vi "GLVT-Main.vi"() -> ()   [LabVIEW 2020]
uses:
  Controls/GLVT-States.ctl
  Controls/GLVT-Stepper-EnableState.ctl
  Controls/GLVT-Stepper-RotateDirection.ctl
  <vilib>/numeric/Random Number (Range) DBL.vi
  Controls/GLVT-FGV-States.ctl
panel:
  out "Filename DTS":string
  out "Save Data Location":path
  in  "Filename Descriptor":string
  out "End Data Collection":bool
  out "Current Angle Array Location":i32
  out "Working":bool
  in  "Measure Valve Button":bool
  out "Collected Data":cluster{dbl[], dbl[]}(graph)
  out "Angles for Data Collection (deg abs)":dbl[](array[numeric])
  in  "Angle per Step":dbl=1.0 min=1.0 step=0.1
  in  "Max Angle to Rotate (deg abs)":dbl
  in  "Pulse Rate (pps)":i32=600
  in  "Steps per Rev":i32=1600
  in  "Move Stepper Button":bool
  in  "Angle to Rotate  (deg abs)":dbl step=0.1
  out "Motor Position Actual":dbl format="%#.2f"
  in  "Release Motor Button":bool
  in  "Motor State":T1
  # "Configuration Only\nDo Not Change"
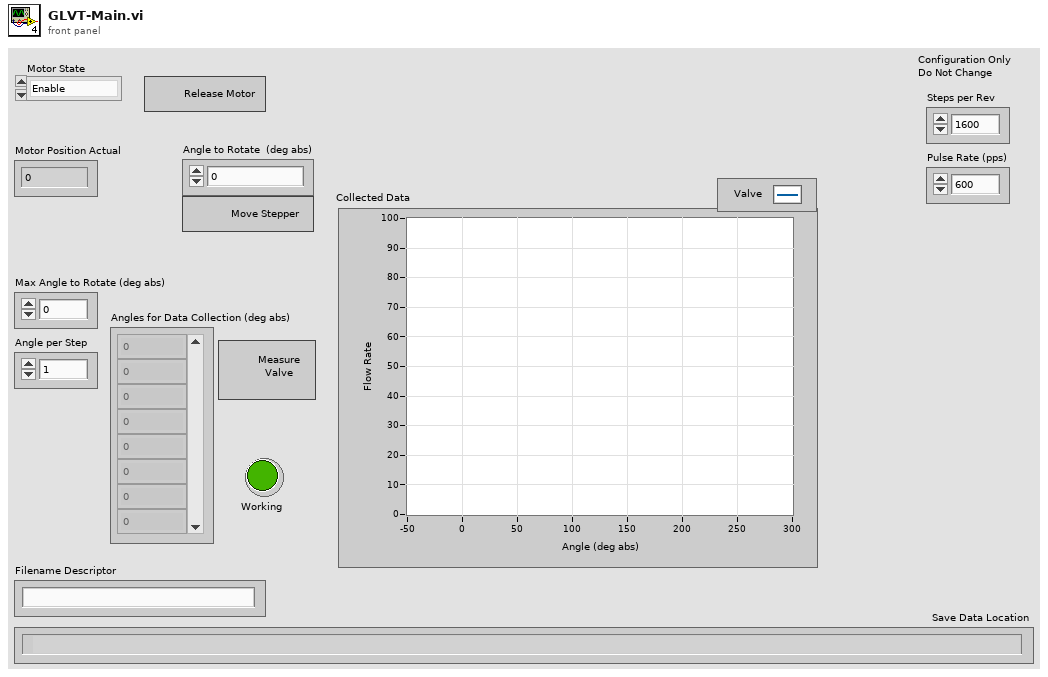
[diagram p1: front panel]
types:
  T1 = typedef "GLVT-Stepper-EnableState.ctl" = enum16{"Enable", "Disable"}
  T2 = typedef "GLVT-States.ctl" = enum16{"Idle", "Initialize", "Read Data", "Next Valve Pos", "Rotate Valve", "Save Data", "Exit"}
  T3 = typedef "GLVT-Stepper-RotateDirection.ctl" = enum16{"CCW", "CW"}
  T4 = typedef "GLVT-FGV-States.ctl" = enum16{"Get", "Set"}
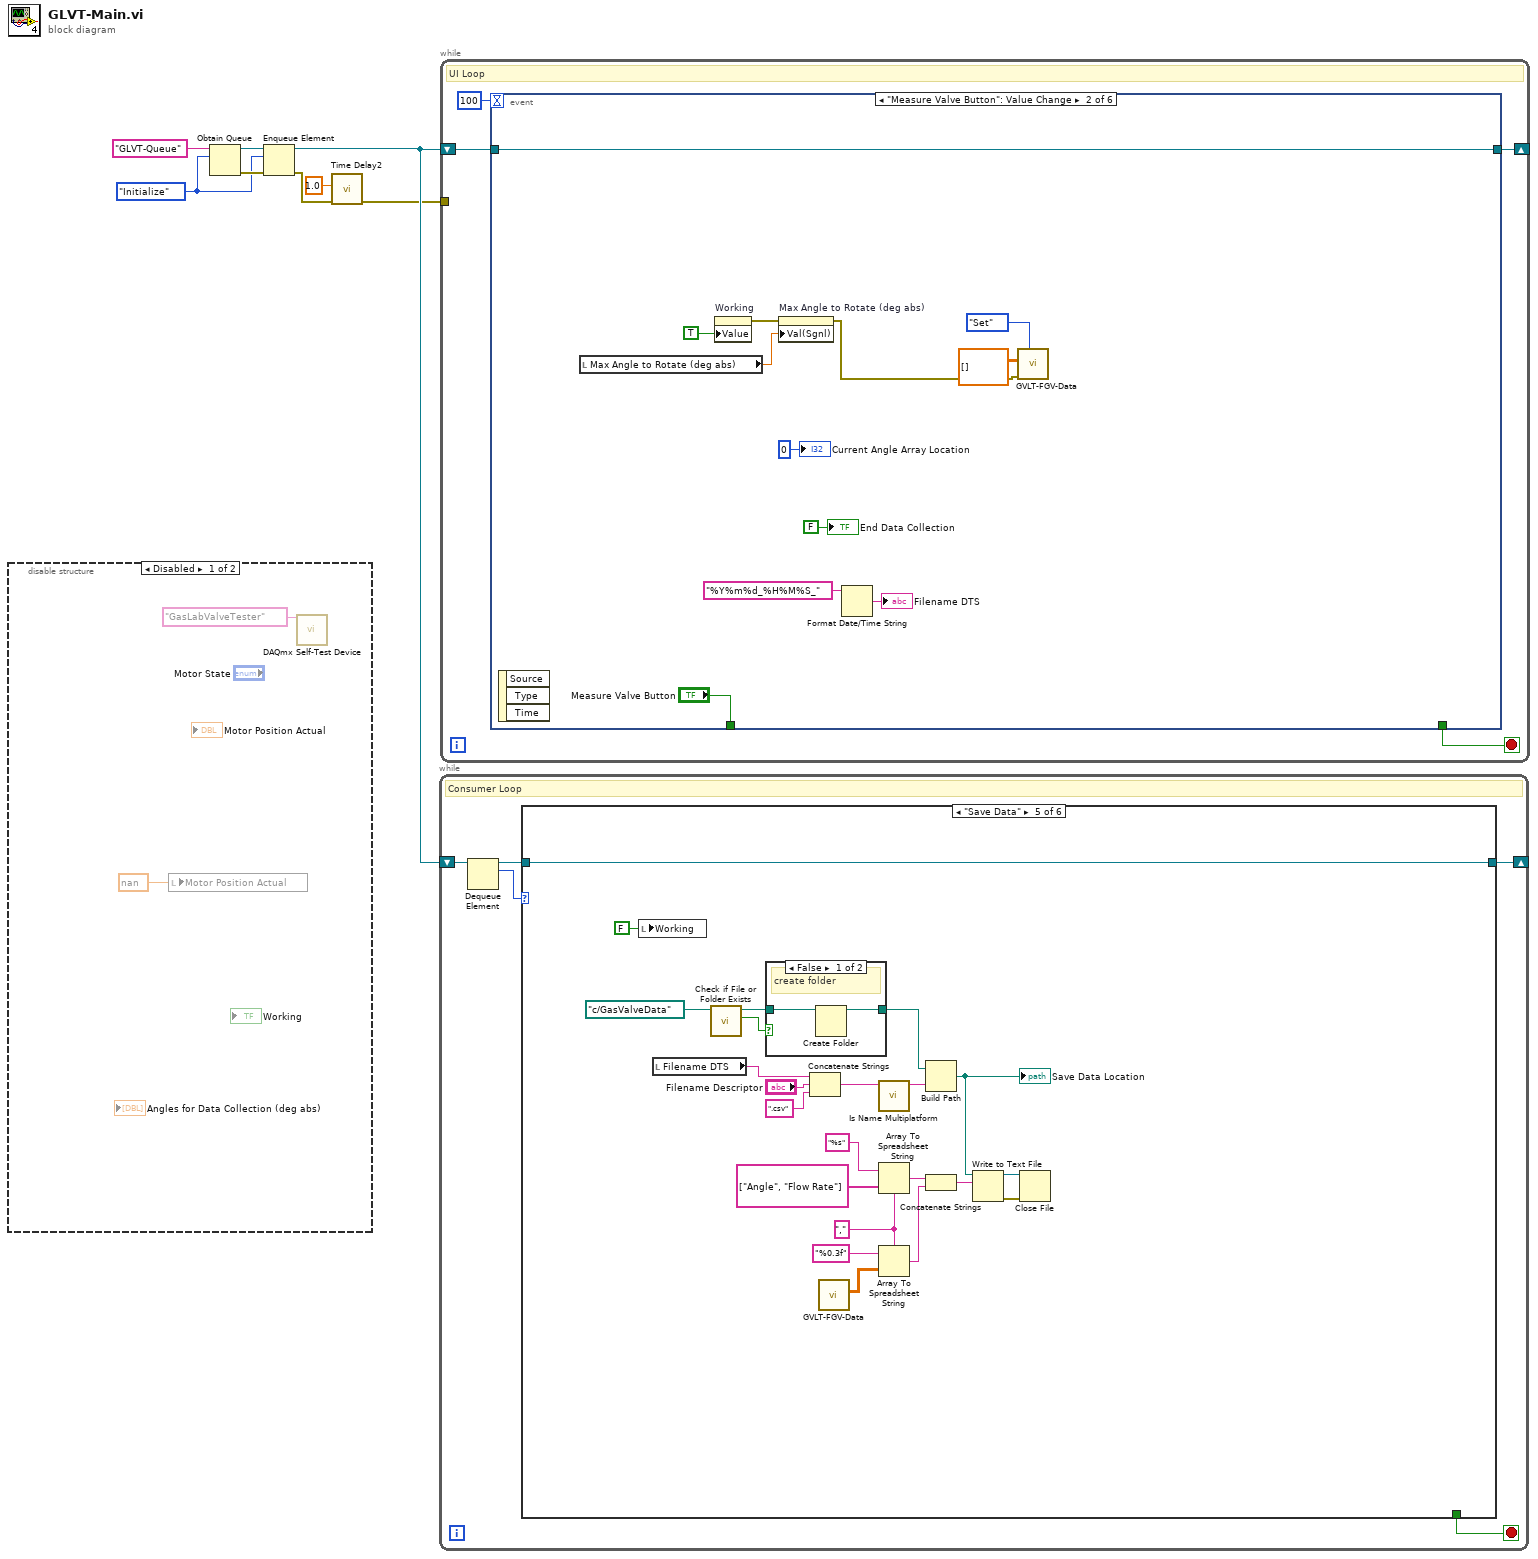
[diagram p0: block diagram]
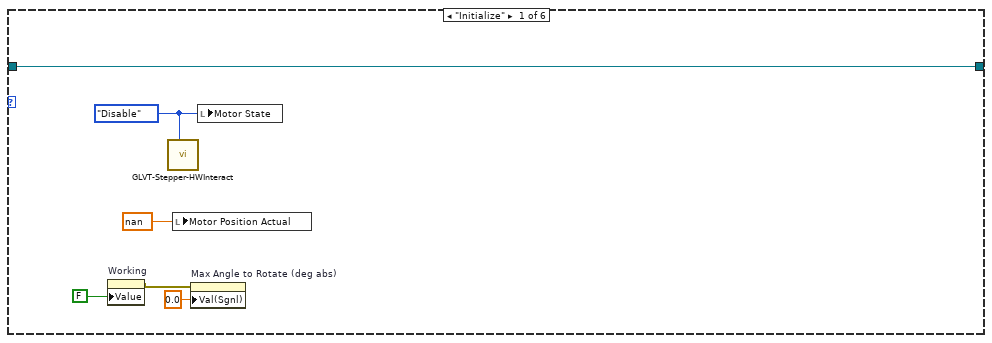
[diagram p3: hidden frame]
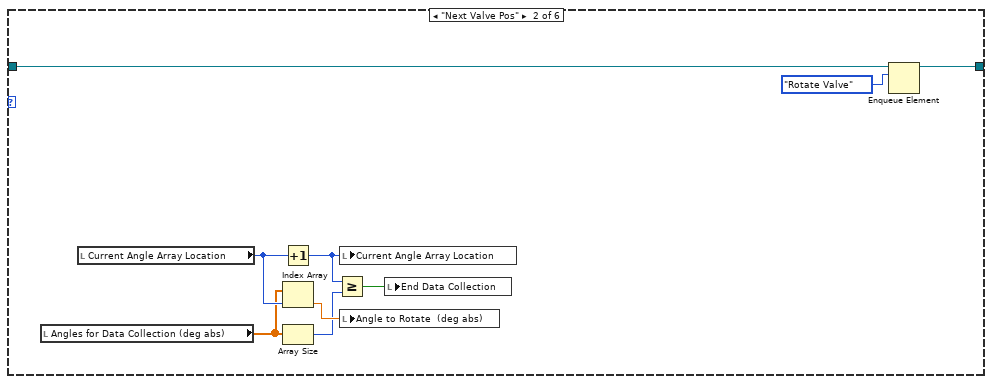
[diagram p4: hidden frame]
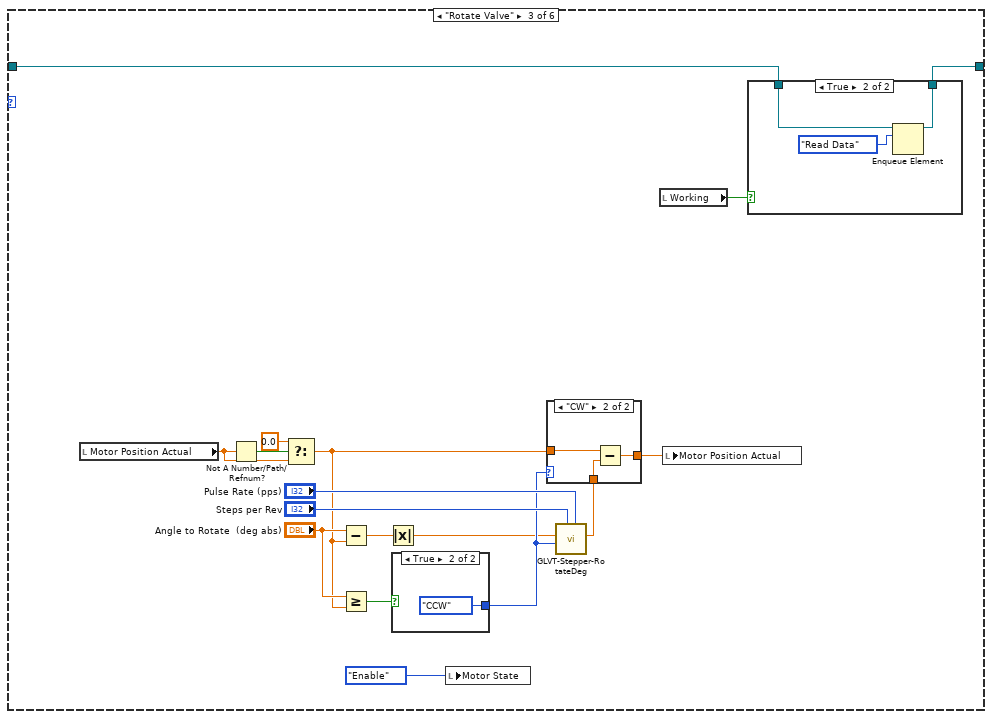
[diagram p5: hidden frame]
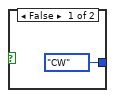
[diagram p7: hidden frame]
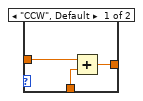
[diagram p8: hidden frame]
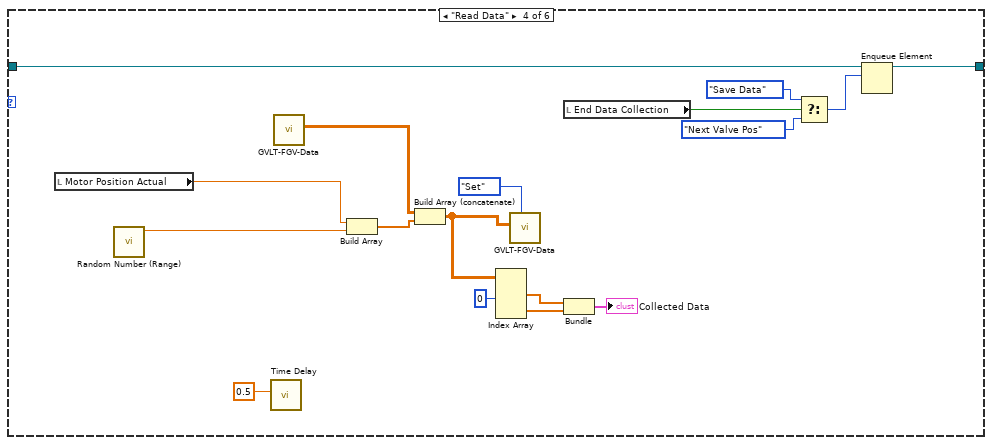
[diagram p9: hidden frame]
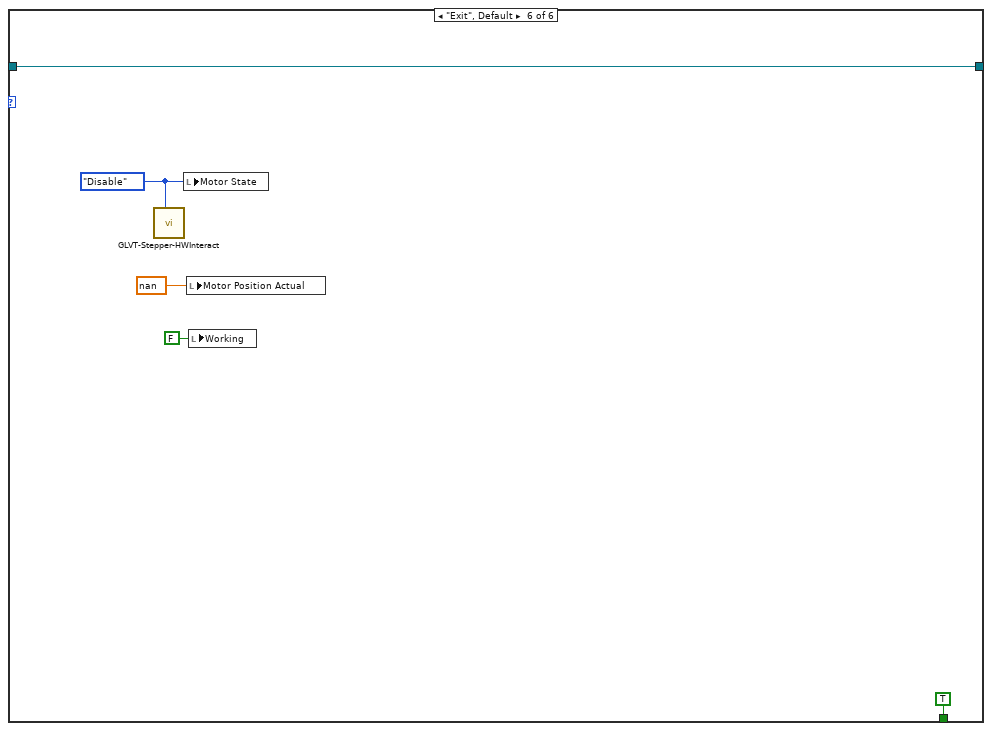
[diagram p11: hidden frame]
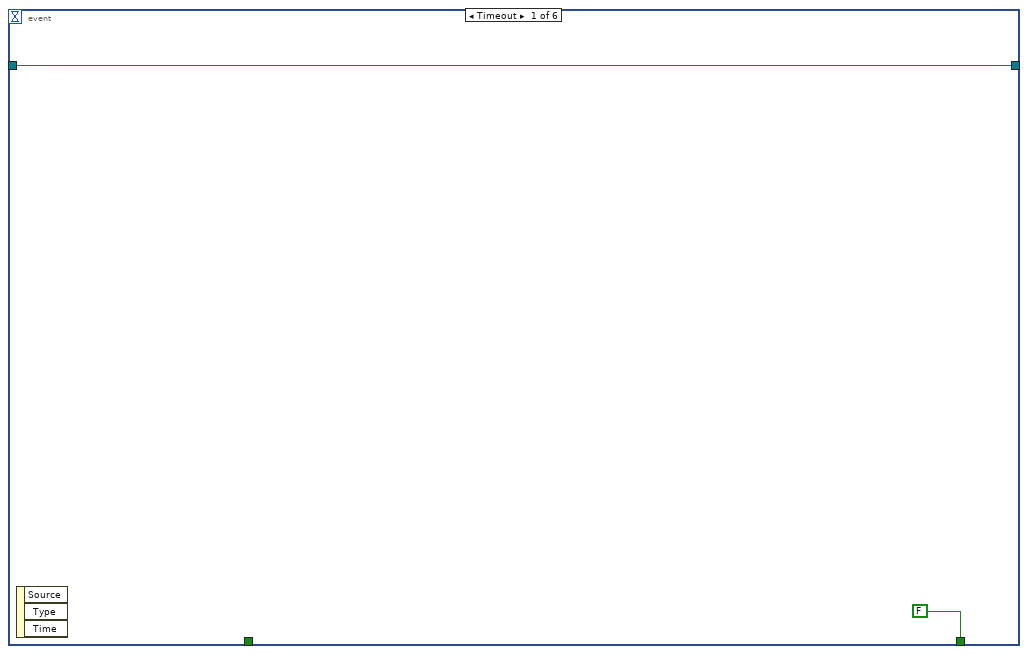
[diagram p12: hidden frame]
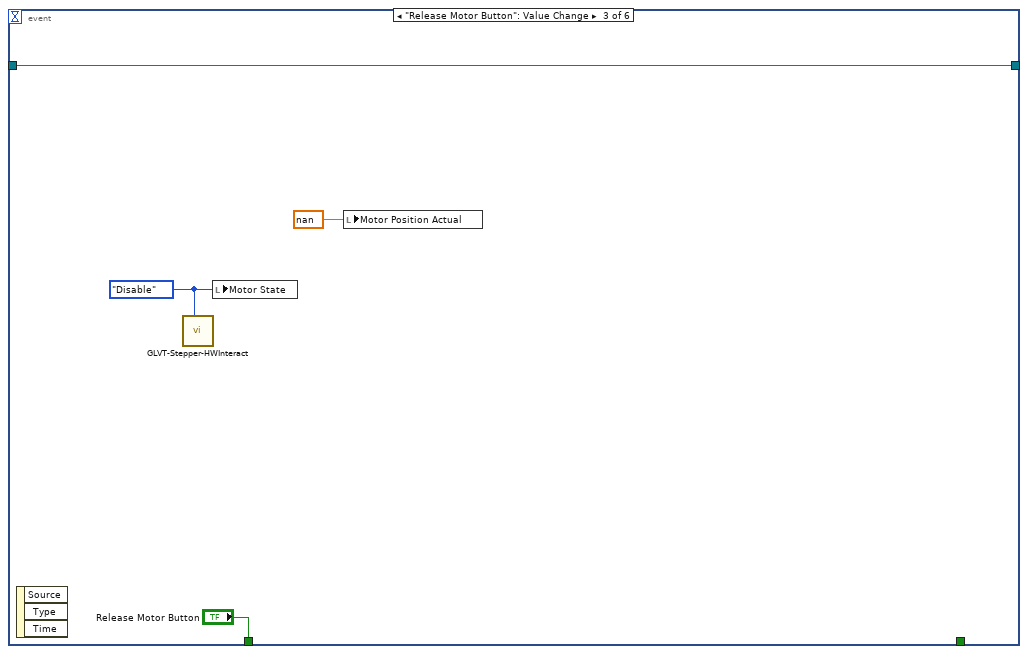
[diagram p13: hidden frame]
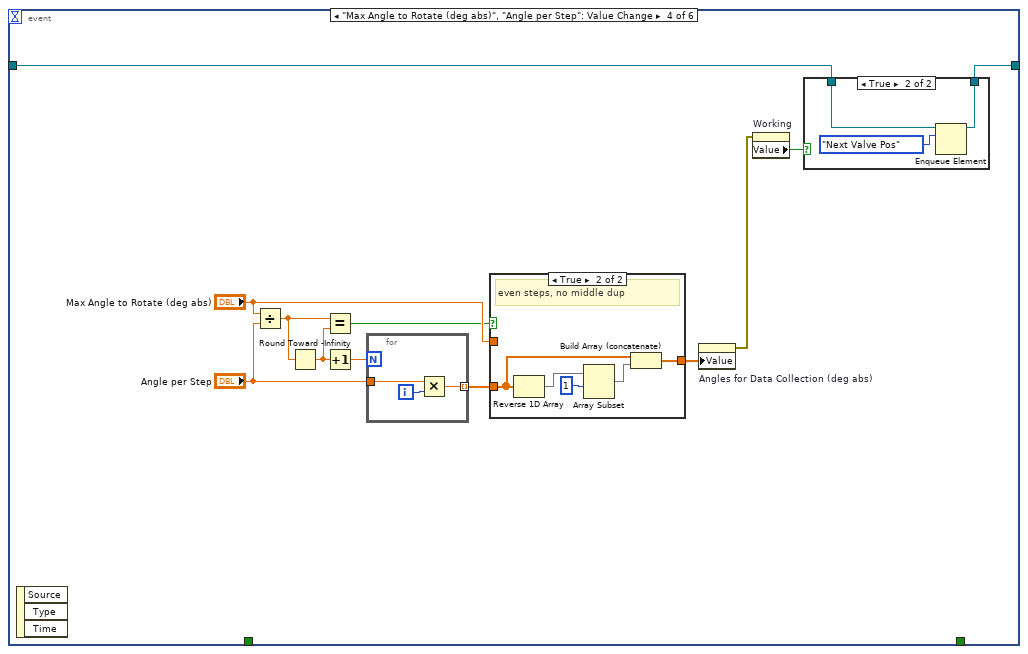
[diagram p14: hidden frame]
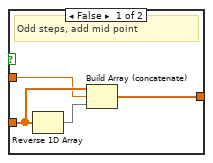
[diagram p16: hidden frame]
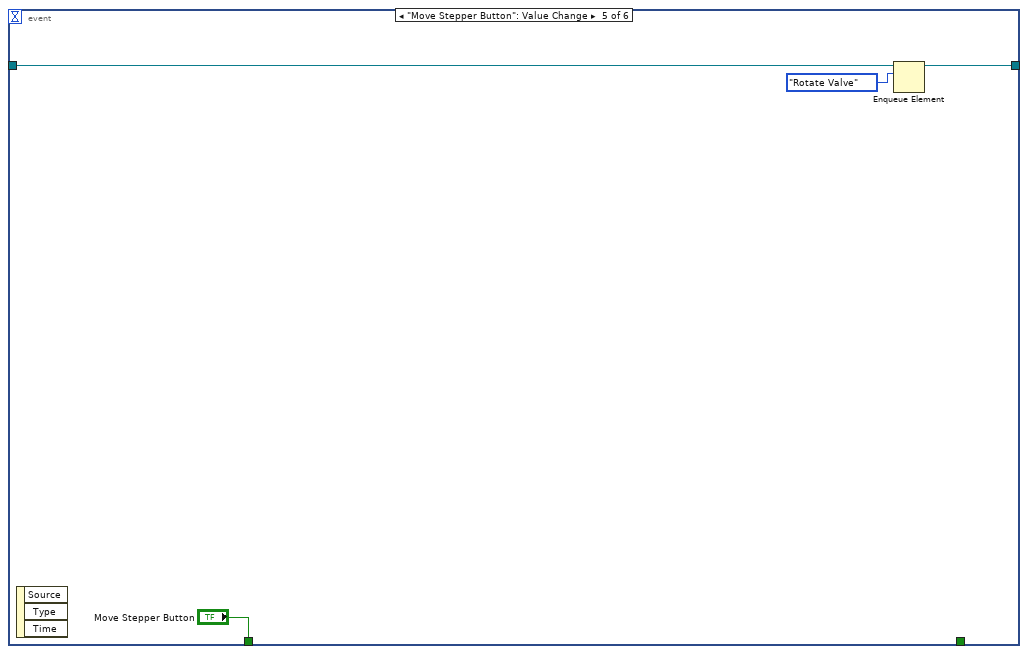
[diagram p17: hidden frame]
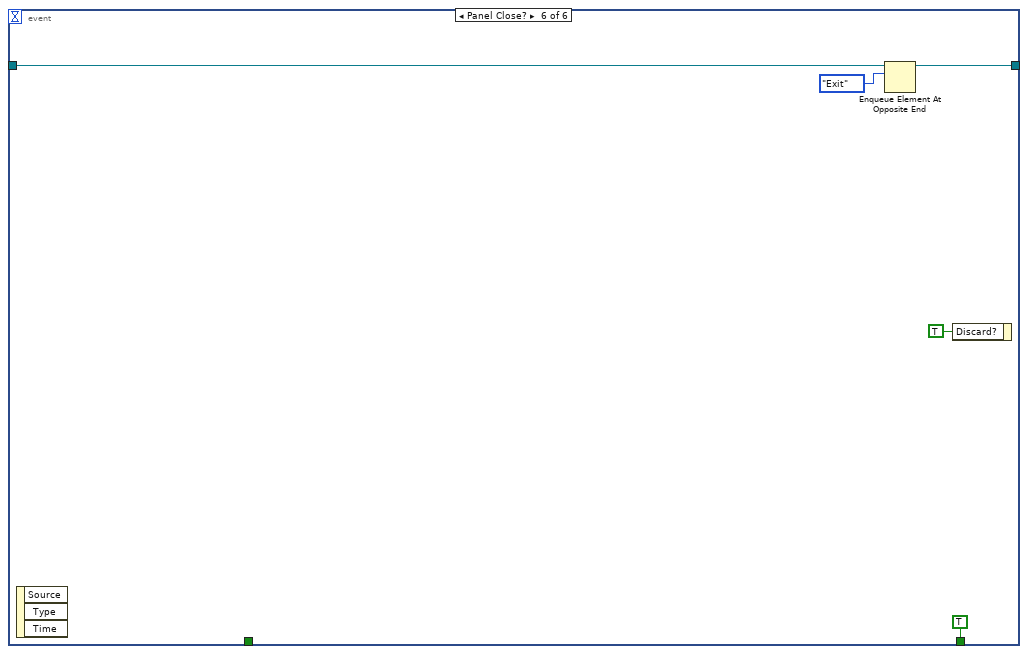
[diagram p18: hidden frame]
diagram:
  w5 = GLVT-States."Initialize"
  n1 = disable-structure shown="Disabled" {
    frame Disabled {
      n2 = local write "Motor Position Actual"(nan ("Motor Position")) -> ()
      n3 = call <vilib>:"DAQmx Self-Test Device.vi"("device in"=tag "GasLabValveTester") -> ()  [unwired: 14 in, 1 out]
    }
    frame Enabled {
    }
  }
  n4 = Obtain Queue(name (unnamed)="GLVT-Queue", element data type=w5) -> (queue out=w6:refnum<queue>, error out=w7:errorcluster)  [unwired: 3 in, 1 out]
  n5 = Enqueue Element(queue=w6, element=w5, error in (no error)=w7) -> (queue out=w4:refnum<queue>, error out=w3:errorcluster)  [unwired: 1 in, 1 out]
  n6 = call "Time Delay2"("error in (no error)"=w3, "Delay Time (s)"=1.0) -> ("error out"=w2:errorcluster)  [unwired: 9 in]
  n7 = while {
    shift-right: [w11] -> _
    shift-left: w4 -> [w14]
    stop <- w15 stop-if-true
    # "Consumer Loop"
    n8 = Dequeue Element(queue=w14) -> (queue out=w13:refnum<queue>, element=w12:T2)  [unwired: 2 in, 2 out]
    n9 = case shown="\"Save Data\"" w12 {
      tunnel: [_ _ _ _ _ TRUE] -> w15
      tunnel: w13 -> [w21 w30 w32 w76 w98 w105]
      tunnel: [w21 w23 w31 w75 w98 w105] -> w11
      frame "Initialize" {
        w20 = GLVT-Stepper-EnableState."Disable" ("GLVT-Enable State")
        n10 = property on="Working" class="Bool (strict)"("Value"=FALSE ("Working")) -> (error out=w16:errorcluster)  [unwired: 2 in, 1 out]
        n11 = call "GLVT-Stepper-HWInteract.vi"("GLVT-Enable State"=w20) -> ()  [unwired: 10 in, 1 out]
        n12 = local write "Motor Position Actual"(nan ("Motor Position")) -> ()
        n13 = property on="Max Angle to Rotate (deg abs)" class="DigNum (strict)"(error in=w16, "Val(Sgnl)"=0.0 ("Value (Signaling)")) -> ()  [unwired: 1 in, 2 out]
        n14 = local write "Motor State"(w20) -> ()
      }
      frame "Next Valve Pos" {
        n15 = local read "Angles for Data Collection (deg abs)"() -> (w27:dbl[])
        n16 = local read "Current Angle Array Location"() -> (w29:i32)
        n17 = Increment(x=w29) -> (x+1=w25:i32)
        n18 = Index Array(array=w27, index=w29) -> (element=w28:dbl)
        n19 = Array Size(array=w27) -> (size(s)=w26:i32)
        n20 = Greater Or Equal?(x=w25, y=w26) -> (x >= y?=w24:bool)
        n21 = local write "Current Angle Array Location"(w25) -> ()
        n22 = local write "Angle to Rotate  (deg abs)"(w28) -> ()
        n23 = local write "End Data Collection"(w24) -> ()
        n24 = Enqueue Element(queue=w30, element=GLVT-States."Rotate Valve") -> (queue out=w23:refnum<queue>)  [unwired: 2 in, 2 out]
      }
      frame "Rotate Valve" {
        n25 = local read "Motor Position Actual"() -> (w41:dbl)
        n26 = Not A Number/Path/Refnum?(number/path/refnum=w41) -> (NaN/Path/Refnum?=w42:bool)
        n27 = Select(t=0.0, s=w42, f=w41) -> (s? t:f=w37:dbl)
        n28 = Subtract(x="Angle to Rotate  (deg abs)", y=w37) -> (x-y=w36:dbl)
        n29 = Greater Or Equal?(x="Angle to Rotate  (deg abs)", y=w37) -> (x >= y?=w40:bool)
        n30 = Absolute Value(x=w36) -> (abs(x)=w35:dbl)
        n31 = case shown="True" w40 {
          tunnel: [GLVT-Stepper-RotateDirection."CW" ("Rotate Direction") GLVT-Stepper-RotateDirection."CCW" ("Rotate Direction")] -> w39
          frame False {
          }
          frame True {
          }
        }
        n32 = local write "Motor State"(GLVT-Stepper-EnableState."Enable" ("GLVT-Enable State")) -> ()
        n33 = call "GLVT-Stepper-RotateDeg.vi"("Pulse Rate (pps)"="Pulse Rate (pps)", "Steps per Rev"="Steps per Rev", "Rotate Direction"=w39, "Rotation Angle (deg)"=w35) -> ("Actual Rotation Angle (deg)"=w47:dbl)  [unwired: 6 in, 1 out]
        n34 = case shown="\"CW\"" w39 {
          tunnel: w37 -> [w56 w59]
          tunnel: w47 -> [w55 w58]
          tunnel: [w54 w57] -> w34
          frame "CCW", Default {
            n35 = Add(x=w56, y=w55) -> (x+y=w54:dbl)
          }
          frame "CW" {
            n36 = Subtract(x=w59, y=w58) -> (x-y=w57:dbl)
          }
        }
        n37 = local read "Working"() -> (w33:bool)
        n38 = local write "Motor Position Actual"(w34) -> ()
        n39 = case shown="True" w33 {
          tunnel: [w48 w50] -> w31
          tunnel: w32 -> [w48 w51]
          frame False {
          }
          frame True {
            n40 = Enqueue Element(queue=w51, element=GLVT-States."Read Data") -> (queue out=w50:refnum<queue>)  [unwired: 2 in, 2 out]
          }
        }
      }
      frame "Read Data" {
        n41 = local read "Motor Position Actual"() -> (w70:dbl)
        n42 = call-poly <vilib>:"Random Number (Range).vi"() -> ("number"=w69:dbl)  [unwired: 11 in]
        n43 = call "Time Delay"("Delay Time (s)"=0.5) -> ()  [unwired: 10 in, 1 out]
        n44 = call "GVLT-FGV-Data.vi"() -> ("Data Out"=w68:dbl[][])  [unwired: 10 in, 1 out]
        n45 = Build Array(w70, w69) -> (w67:dbl[])
        n46 = Build Array (concatenate)(w68, w67) -> (w65:dbl[][])
        n47 = Index Array(array=w65, index (col) #1=0 ("disabled index (col)")) -> (element #1=w63:dbl[], element #2=w62:dbl[])  [unwired: 3 in]
        n48 = call "GVLT-FGV-Data.vi"("State"=GLVT-FGV-States."Set", "Data In"=w65) -> ()  [unwired: 8 in, 2 out]
        n49 = local read "End Data Collection"() -> (w74:bool)
        n50 = Bundle(w63, w62) -> (→"Collected Data":cluster{dbl[], dbl[]})  [unwired: 1 in]
        n51 = Select(t=GLVT-States."Save Data" ("element"), s=w74, f=GLVT-States."Next Valve Pos" ("element")) -> (s? t:f=w71:T2)
        n52 = Enqueue Element(queue=w76, element=w71) -> (queue out=w75:refnum<queue>)  [unwired: 2 in, 2 out]
      }
      frame "Save Data" {
        w86 = "," ("delimiter (Tab)")
        n53 = local write "Working"(FALSE ("Working")) -> ()
        n54 = local read "Filename DTS"() -> (w95:string)
        n55 = call <vilib>:"Check if File or Folder Exists.vi"("path"=path "c:/GasValveData") -> ("file or folder exists?"=w91:bool, "dup path"=w90:path)  [unwired: 8 in, 1 out]
        n56 = case shown="False" w91 {
          tunnel: w90 -> [w100 w101]
          tunnel: [w99 w101] -> w82
          frame False {
            # "create folder"
            n57 = Create Folder(path (use dialog)=w100) -> (created path=w99:path)  [unwired: 2 in, 2 out]
          }
          frame True {
            # "exists, do nothing"
          }
        }
        n58 = Concatenate Strings(w95, "Filename Descriptor", ".csv" ("string")) -> (w93:string)
        n59 = call "GVLT-FGV-Data.vi"() -> ("Data Out"=w89:dbl[][])  [unwired: 10 in, 1 out]
        n60 = call <vilib>:"Is Name Multiplatform.vi"("filename"=w93) -> ("suggested filename"=w81:string)  [unwired: 6 in, 4 out]
        n61 = Array To Spreadsheet String(delimiter (Tab)=w86, array=string[] ["Angle", "Flow Rate"], 3:"%s" ("format string")) -> (spreadsheet string=w84:string)
        n62 = Array To Spreadsheet String(delimiter (Tab)=w86, array=w89, 3:"%0.3f" ("format string")) -> (spreadsheet string=w83:string)
        n63 = Build Path(base path=w82, name or relative path=w81) -> (appended path=w77:path)
        "Save Data Location" <- w77
        n64 = Concatenate Strings(w84, w83) -> (w80:string)
        n65 = Write to Text File(file (use dialog)=w77, text=w80) -> (refnum out=w78:refnum<file>, error out=w79:errorcluster)  [unwired: 2 in, 1 out]
        n66 = Close File(refnum=w78, error in=w79) -> ()  [unwired: 2 out]
      }
      frame "Exit", Default {
        w104 = GLVT-Stepper-EnableState."Disable" ("GLVT-Enable State")
        n67 = call "GLVT-Stepper-HWInteract.vi"("GLVT-Enable State"=w104) -> ()  [unwired: 10 in, 1 out]
        n68 = local write "Motor State"(w104) -> ()
        n69 = local write "Motor Position Actual"(nan ("Motor Position")) -> ()
        n70 = local write "Working"(FALSE ("Working")) -> ()
      }
    }
  }
  n71 = while {
    shift-right: [w107] -> _
    shift-left: w4 -> [w108]
    tunnel: w2 -> [_]
    stop <- w110 stop-if-true
    # "UI Loop"
    n72 = event shown="[1] \"Measure Valve Button\": Value Change" {
      selector: _ -> [_ _ _ _ _ _]
      dyn-events: _ -> [_ _ _ _ _ _]
      timeout: 100 -> [_ _ _ _ _ _]
      tunnel: [FALSE _ _ _ _ TRUE] -> w110
      tunnel: w108 -> [w111 w124 w128 w130 w160 w165]
      tunnel: [w111 w124 w128 w129 w158 w162] -> w107
      tunnel: [_ "Measure Valve Button" "Release Motor Button" _ "Move Stepper Button" _] -> _
      event Timeout {
        n73 = event-data() -> ()  [unwired: 1 in, 3 out]
      }
      event "Measure Valve Button": Value Change {
        n74 = event-data() -> ()  [unwired: 1 in, 3 out]
        n75 = local read "Max Angle to Rotate (deg abs)"() -> (w122:dbl)
        n76 = property on="Working" class="Bool (strict)"("Value"=TRUE ("Working")) -> (error out=w120:errorcluster)  [unwired: 2 in, 1 out]
        n77 = property on="Max Angle to Rotate (deg abs)" class="DigNum (strict)"(error in=w120, "Val(Sgnl)"=w122) -> (error out=w115:errorcluster)  [unwired: 1 in, 1 out]
        n78 = Format Date/Time String(time format string (%c)="%Y%m%d_%H%M%S_") -> (date/time string=→"Filename DTS":string)  [unwired: 2 in]
        n79 = call "GVLT-FGV-Data.vi"("State"=GLVT-FGV-States."Set", "error in"=w115, "Data In"=dbl[][] []) -> ()  [unwired: 7 in, 2 out]
        "Current Angle Array Location" <- 0 ("Current Angle Array Location")
        "End Data Collection" <- FALSE ("End Data Collection")
      }
      event "Release Motor Button": Value Change {
        w126 = GLVT-Stepper-EnableState."Disable" ("GLVT-Enable State")
        n80 = event-data() -> ()  [unwired: 1 in, 3 out]
        n81 = call "GLVT-Stepper-HWInteract.vi"("GLVT-Enable State"=w126) -> ()  [unwired: 10 in, 1 out]
        n82 = local write "Motor State"(w126) -> ()
        n83 = local write "Motor Position Actual"(nan ("Motor Position")) -> ()
      }
      event "Max Angle to Rotate (deg abs)", "Angle per Step": Value Change {
        n84 = event-data() -> ()  [unwired: 1 in, 3 out]
        n85 = Divide(x="Max Angle to Rotate (deg abs)", y="Angle per Step") -> (x/y=w136:dbl)
        n86 = Round Toward -Infinity(1:w136) -> (0:w135:dbl)
        n87 = Equal?(x=w136, y=w135) -> (x = y?=w134:bool)
        n88 = Increment(x=w135) -> (x+1=w140:dbl)
        n89 = for {
          N: w140 -> [_]
          tunnel: "Angle per Step" -> [w155]
          tunnel: [w154] -> w138 mode=indexing
          i -> [w156]
          n90 = Multiply(x=w155, y=w156) -> (x*y=w154:dbl)
        }
        n91 = case shown="True" w134 {
          tunnel: [w148 w149] -> w133
          tunnel: w138 -> [w147 w150]
          tunnel: "Max Angle to Rotate (deg abs)" -> [w145 _]
          frame False {
            # "Odd steps, add mid point"
            n92 = Reverse 1D Array(array=w147) -> (reversed array=w146:dbl[])
            n93 = Build Array (concatenate)(w147, w145, w146) -> (w148:dbl[])
          }
          frame True {
            # "even steps, no middle dup"
            n94 = Reverse 1D Array(array=w150) -> (reversed array=w153:dbl[])
            n95 = Array Subset(array=w153, index=1) -> (w151:dbl[])  [unwired: 1 in]
            n96 = Build Array (concatenate)(w150, w151) -> (w149:dbl[])
          }
        }
        n97 = property on="Angles for Data Collection (deg abs)" class="Arr (strict)"("Value"=w133) -> (error out=w132:errorcluster)  [unwired: 2 in, 1 out]
        n98 = property on="Working" class="Bool (strict)"(error in=w132) -> ("Value"=w131:bool)  [unwired: 1 in, 2 out]
        n99 = case shown="True" w131 {
          tunnel: [w141 w143] -> w129
          tunnel: w130 -> [w141 w144]
          frame False {
          }
          frame True {
            n100 = Enqueue Element(queue=w144, element=GLVT-States."Next Valve Pos") -> (queue out=w143:refnum<queue>)  [unwired: 2 in, 2 out]
          }
        }
      }
      event "Move Stepper Button": Value Change {
        n101 = event-data() -> ()  [unwired: 1 in, 3 out]
        n102 = Enqueue Element(queue=w160, element=GLVT-States."Rotate Valve") -> (queue out=w158:refnum<queue>)  [unwired: 2 in, 2 out]
      }
      event Panel Close? {
        n103 = event-data() -> ()  [unwired: 1 in, 3 out]
        n104 = Enqueue Element At Opposite End(queue=w165, element=GLVT-States."Exit") -> (queue out=w162:refnum<queue>)  [unwired: 2 in, 2 out]
        n105 = event-data("Discard?"=TRUE) -> ()  [unwired: 1 in, 1 out]
      }
    }
  }
